vi "Authenticate SSL Server.vi"(8 "Error In":errorcluster, 9 "Input Data":T1 {"Ssl Protocols Type" items=["None"=0, "Ssl2"=12, "Ssl3"=48, "Tls"=192, "Default"=240]}, 11 "SSL Stream":refnum<k24>) -> (0 "Error Out":errorcluster)   [LabVIEW 2014, in "SSL Lib.lvlib"]
doc: "VI Function: This VI is called by the server to authenticate the server and optionally the client in a Clinet-Server connection.\n\nVI Version: 1.0\n\nVI Author: Runjhun Agarwal"
uses:
  <userlib>/SSL Library/SSL Lib.lvlib
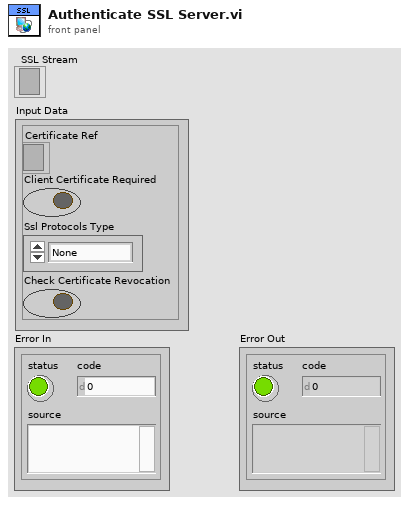
[diagram p1: front panel]
types:
  T1 = cluster{"Certificate Ref":refnum<k24>, "Client Certificate Required":bool, "Ssl Protocols Type":i32, "Check Certificate Revocation":bool}
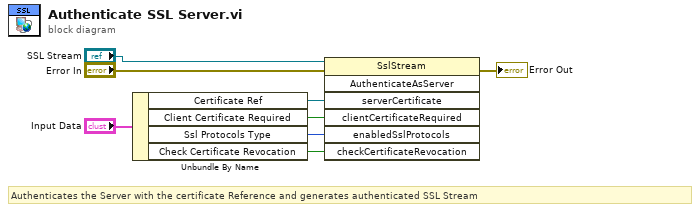
[diagram p0: block diagram]
diagram:
  # "Authenticates the Server with the certificate Reference and generates authenticated SSL Stream"
  n1 = Unbundle By Name("Input Data") -> ("Certificate Ref"=w7:refnum<k24>, "Client Certificate Required"=w6:bool, "Ssl Protocols Type"=w5:i32, "Check Certificate Revocation"=w4:bool)
  n2 = invoke class="SslStream" method="AuthenticateAsServer"(reference="SSL Stream", error in="Error In", "serverCertificate"=w7, "clientCertificateRequired"=w6, "enabledSslProtocols"=w5, "checkCertificateRevocation"=w4) -> (error out=→"Error Out":errorcluster)  [unwired: 1 in, 6 out]
